vi "Navigation_Main_420.vi"() -> ()   [LabVIEW 2015]
uses:
  <vilib>/myRIO/Instrument Drivers/Onboard IO/PWM/typedefs/PWM Reference.ctl
  <vilib>/myRIO/Common/Instrument Driver Framework/Utilities/typedefs/myRIO Generic Hardware Reference.ctl
  <vilib>/myRIO/Common/Instrument Driver Framework/Utilities/typedefs/Hardware Version Enum.ctl
  <vilib>/myRIO/Common/Instrument Driver Framework/Utilities/typedefs/myRIO v1.0 Reference.ctl
  <vilib>/myRIO/Common/Instrument Driver Framework/Utilities/typedefs/Generic FPGA Reference.ctl
  <vilib>/myRIO/Common/Instrument Driver Framework/myRIO v1.0/PWM/typedefs/PWM Channels Enum.ctl
  <vilib>/myRIO/Instrument Drivers/Onboard IO/PWM/typedefs/PWM Configuration.ctl
  <vilib>/userdefined/High Color/nirio_resource_hc.ctl
  <vilib>/myRIO/Common/Instrument Driver Framework/myRIO v1.0/PWM/vis/myRIO v1.1 Open PWM.vi
  <vilib>/myRIO/Common/Instrument Driver Framework/Utilities/vis/Validate Channels.vi
  <vilib>/myRIO/Common/Instrument Driver Framework/myRIO v1.0/PWM/vis/myRIO v1.0 Reserve PWM.vi
  <vilib>/myRIO/Common/Instrument Driver Framework/myRIO v1.0/PWM/vis/myRIO v1.0 Build MUX Configuration PWM.vi
  <vilib>/myRIO/Common/Instrument Driver Framework/myRIO v1.0/Resource Manager/vis/myRIO v1.0 Reserve Channel List.vi
  <vilib>/myRIO/Common/Instrument Driver Framework/myRIO v1.0/Resource Manager/vis/myRIO v1.0 Create Configuration List.vi
  <vilib>/myRIO/Common/Instrument Driver Framework/myRIO v1.0/Resource Manager/vis/myRIO v1.0 Reserve Channel.vi
  <vilib>/myRIO/Common/Instrument Driver Framework/myRIO v1.0/Resource Manager/vis/myRIO v1.0 Unreserve Channel.vi
  <vilib>/myRIO/Common/Instrument Driver Framework/myRIO v1.0/Resource Manager/vis/myRIO v1.0 Build Mutex Name.vi
  <vilib>/FPGAPlugInAG/myRIO-1900/niLvFpga_Open_myRIO-1900.vi
  <vilib>/rvi/interface/common/dynamic/niFpgaDynamicAddResources.vi
  <vilib>/myRIO/Common/Instrument Driver Framework/Utilities/vis/FPGA Ref Manager.vi
  <vilib>/Utility/error.llb/Error Cluster From Error Code.vi
  <vilib>/myRIO/Common/Instrument Driver Framework/Utilities/vis/Ref Counter.vi
  <vilib>/rvi/errors/niLvFpgaAdjustHostInterfaceError.vi
  <vilib>/Utility/VariantDataType/GetNumericInfo.vi
  <vilib>/myRIO/Common/Instrument Driver Framework/myRIO v1.0/myRIO v1.1 Open.vi
  <vilib>/myRIO/Common/Instrument Driver Framework/Utilities/vis/IO Manager.vi
  <vilib>/myRIO/Common/Instrument Driver Framework/Utilities/vis/Configuration Manager.vi
  <vilib>/myRIO/Common/Instrument Driver Framework/myRIO v1.0/Resource Manager/vis/myRIO v1.0 Configure IO.vi
  <vilib>/myRIO/Common/Instrument Driver Framework/myRIO v1.0/myRIO v1.0 Close.vi
  <vilib>/myRIO/Common/Instrument Driver Framework/myRIO v1.0/PWM/vis/myRIO v1.0 Write PWM.vi
  <vilib>/addons/control/pid/pid.llb/PID (DBL).vi
  <vilib>/rvi/interface/nirviOpenFPGA/nirviOpenFPGA.xnode
  Navi/E/FPGA Bitfiles/NavigationProjec_FPGATarget2_FPGAMainNavigati_PWPHW8gwDxI.lvbitx
  <vilib>/rvi/interface/nirviReadWriteControl/nirviReadWriteControl.xnode
  <vilib>/myRIO/Instrument Drivers/Onboard IO/PWM/vis/myRIO PWM Open.xnode
  <vilib>/myRIO/Instrument Drivers/Onboard IO/PWM/PWM.lvlib
  <vilib>/myRIO/Instrument Drivers/Utilities/Utilities.lvlib
  NiFpgaLv.dll
  <vilib>/rvi/interface/Simulation/niFpgaSimulationCallBeginRW.vi
  <vilib>/addons/control/pid/NI_PID_pid.lvlib
panel:
  in  "start":dbl
  in  "end mining section":bool
  in  "frame":dbl format="%#_13g"
  in  "goal":dbl=10.0
  in  "first good x":dbl
  in  "drive 1 ft":dbl
  in  "end loop":bool
  out "stop switch":dbl
  in  "camera drop":dbl
  in  "derp":dbl
  in  "dead recon offset":dbl
  in  "last good x":dbl
  out "scale 2":dbl=1.0
  out "distance to goal":dbl
  out "loc_y":dbl
  out "loc_x":dbl
  out "loc_theta":dbl
  out "start y":dbl
  out "start angle":dbl=1.0
  out "start x":dbl=1.0
  in  "set start position":bool
  in  "R Min Linear Velocity (ft/s)  2":dbl=-2.0 format="%#_13g"
  in  "L Min Linear Velocity (ft/s) 9":dbl=-2.0 format="%#_13g"
  in  "R Max Linear Velocity (ft/s) 5":dbl=2.0 format="%#_13g"
  in  "L Max Linear Velocity (ft/s) 5":dbl=2.0 format="%#_13g"
  out "left wheels actual pwm":dbl
  in  "stop 3":bool
  out "left pwm":dbl(graph)
  out "dt out (s) 3":dbl format="%.3f"
  in  "output range 3":cluster{"output high":dbl, "output low":dbl}={"output high"=0.13333, "output low"=-0.13333} {"output low" format="%.6f"; "output high" format="%.5f"}
  in  "PID gains 3":T1={"proportional gain (Kc)"=0.002, "integral time (Ti, min)"=7e-07, "derivative time (Td, min)"=0.0} {"derivative time (Td, min)" format="%.8f"; "integral time (Ti, min)" format="%.8f"; "proportional gain (Kc)" format="%.8f"}
  out "desired pwm 2":dbl
  out "feedback 2":dbl
  out ".not. x? 3":bool
  out "Elapsed Time (s) 2":dbl caption="Elapsed Time (s)"
  out "right wheels actual pwm":dbl
  in  "stop 2":bool
  out "right pwm":dbl(graph)
  out "dt out (s) 2":dbl format="%.3f"
  in  "output range 2":cluster{"output high":dbl, "output low":dbl}={"output high"=0.13333, "output low"=-0.13333} {"output low" format="%.6f"; "output high" format="%.5f"}
  in  "PID gains 2":T1={"proportional gain (Kc)"=0.002, "integral time (Ti, min)"=7e-07, "derivative time (Td, min)"=0.0} {"derivative time (Td, min)" format="%.8f"; "integral time (Ti, min)" format="%.8f"; "proportional gain (Kc)" format="%.8f"}
  out "desired pwm":dbl
  out "feedback":dbl
  out ".not. x? 2":bool
  out "Elapsed Time (s)":dbl
  out "LF Rot Velocity (rot/s)":dbl
  out "LM Rot Velocity (rot/s)":dbl
  out "LR Rot Velocity (rot/s)":dbl
  out "RR Rot Velocity (rot/s)":dbl
  out "RM Linear Velocity (rot/s)":dbl
  out "RF Linear Velocity (rot/s)":dbl
  in  "Encoder Reset":bool
  out "SYS.SELECTA":u8 format="%08b"
  out "ENC.B_c.CNTR":i32
  out "ENC.B_b.CNTR":i32
  out "ENC.B_a.CNTR":i32
  out "ENC.A_c.CNTR":i32
  out "ENC.A_b.CNTR":i32
  out "ENC.A_a.CNTR":i32
  in  "R Min Linear Velocity (ft/s)":dbl=-2.0 format="%#_13g"
  in  "R Max Linear Velocity (ft/s)":dbl=2.0 format="%#_13g"
  in  "L Min Linear Velocity (ft/s)":dbl=-2.0 format="%#_13g"
  in  "L Max Linear Velocity (ft/s)":dbl=2.0 format="%#_13g"
  out "Current Rot Velocity (rot/s)":T2(graph)
  # "Motor Control Parameters"
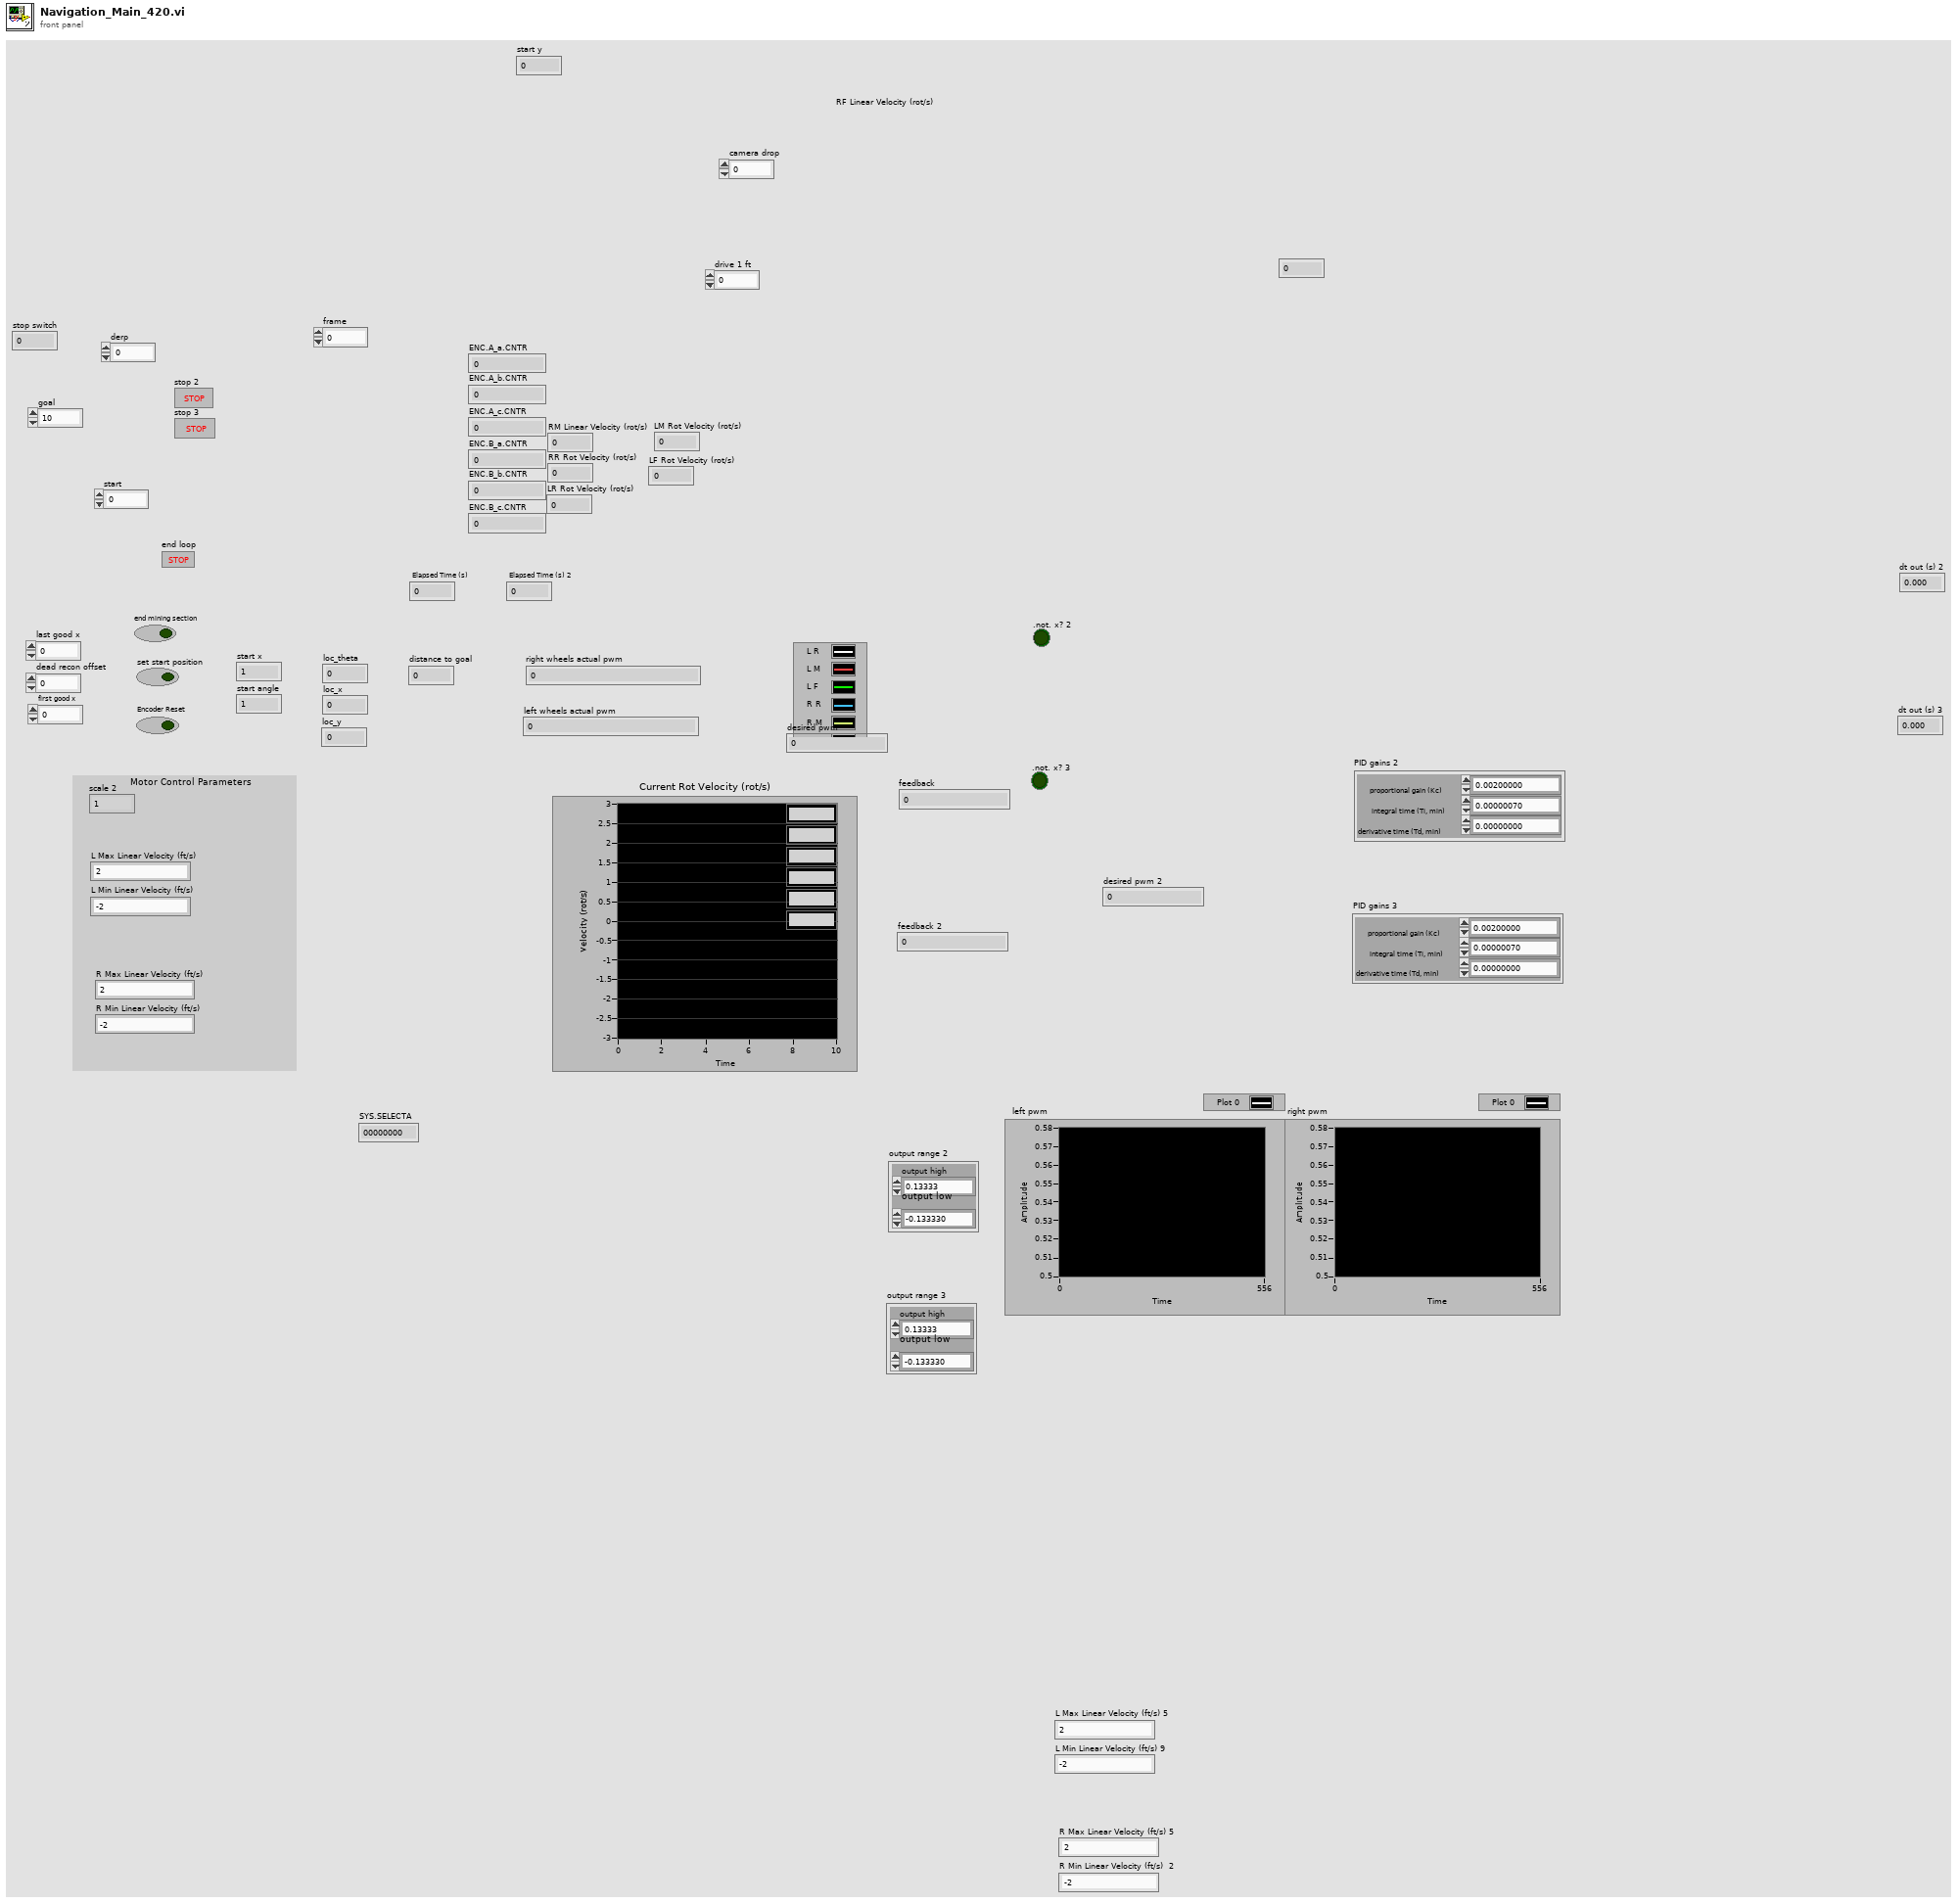
[diagram p1: front panel]
types:
  T1 = cluster{"proportional gain (Kc)":dbl, "integral time (Ti, min)":dbl, "derivative time (Td, min)":dbl}
  T2 = cluster{"Rotational Velocity (RPS)":dbl, "Rotational Velocity (RPS)":dbl, "Rotational Velocity (RPS)":dbl, "Rotational Velocity (RPS)":dbl, "Rotational Velocity (RPS)":dbl, "Rotational Velocity (RPS)":dbl}
  T3 = typedef "nirio_resource_hc.ctl" = tag
  T4 = typedef "Hardware Version Enum.ctl" = enum16{"Unknown", "myRIO-1900", "myRIO-1950", "roboRIO"}
  T5 = typedef "PWM.lvlib/PWM Reference.ctl" = cluster{"myRIO Reference":T6, "PWM Channels Enum":T9, "PWM Configuration":T10}
  T6 = typedef "myRIO Generic Hardware Reference.ctl" = cluster{"myRIO Model":T4, "myRIO Hardware Reference":T7}
  T7 = typedef "myRIO v1.0 Reference.ctl" = cluster{"Generic FPGA Reference":T8, "Allow multiple opens":bool}
  T8 = typedef "Generic FPGA Reference.ctl" = refnum<k20>
  T9 = typedef "PWM Channels Enum.ctl" = enum16{"Not Connected", "C/PWM0", "C/PWM1", "A/PWM0", "A/PWM1", "A/PWM2", "B/PWM0", "B/PWM1", "B/PWM2", "PWM/PWM0", "PWM/PWM1", "PWM/PWM2", "PWM/PWM3", "PWM/PWM4", "PWM/PWM5", "PWM/PWM6", "PWM/PWM7", "PWM/PWM8", "PWM/PWM9"}
  T10 = typedef "PWM.lvlib/PWM Configuration.ctl" = cluster{"Frequency":dbl, "Duty Cycle":dbl}
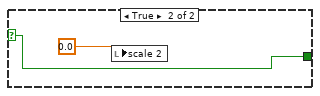
[diagram p3: hidden frame]
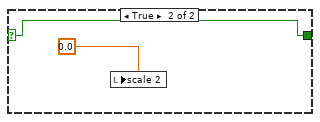
[diagram p4: hidden frame]
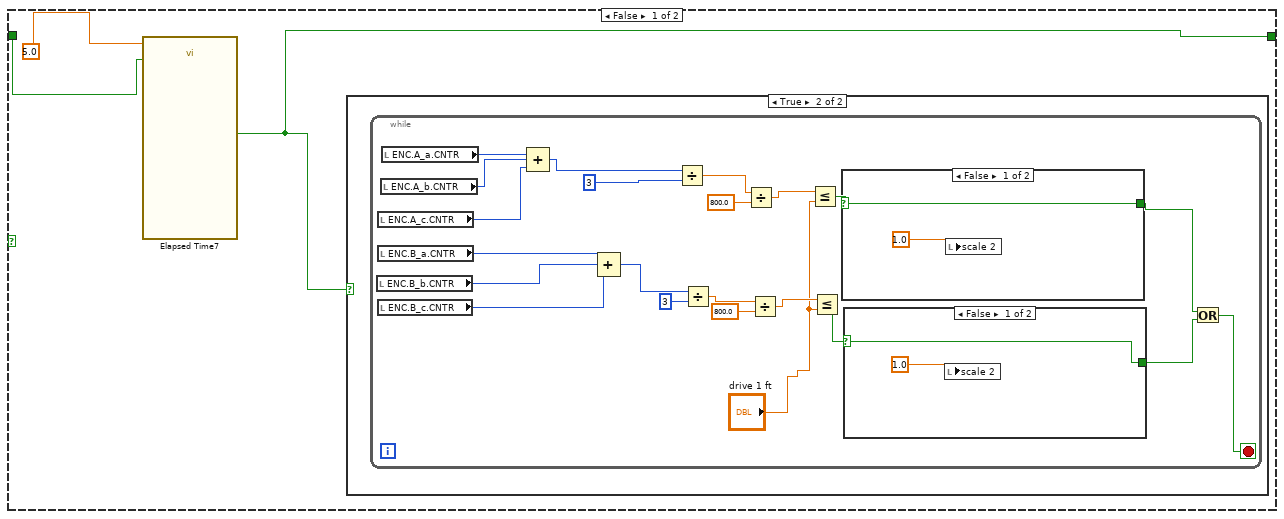
[diagram p5: hidden frame]
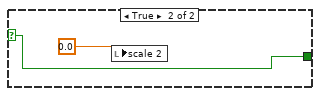
[diagram p7: hidden frame]
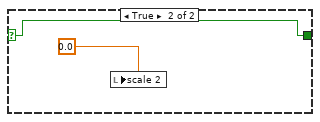
[diagram p8: hidden frame]
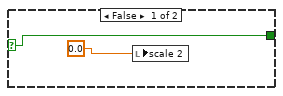
[diagram p9: hidden frame]
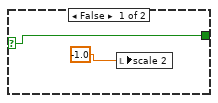
[diagram p10: hidden frame]
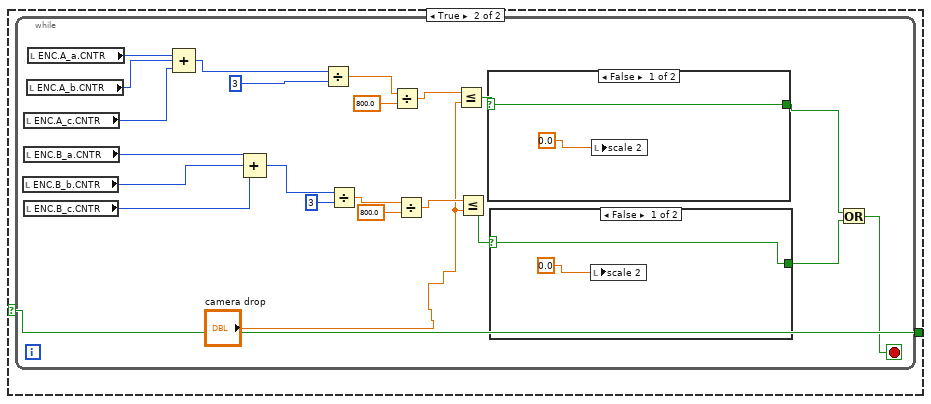
[diagram p11: hidden frame]
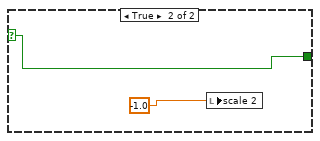
[diagram p12: hidden frame]
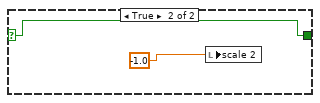
[diagram p13: hidden frame]
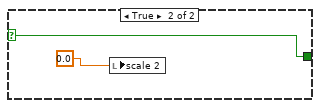
[diagram p14: hidden frame]
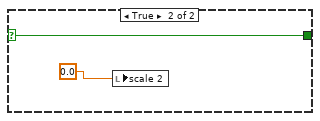
[diagram p15: hidden frame]
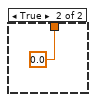
[diagram p17: hidden frame]
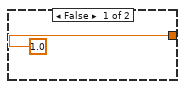
[diagram p18: hidden frame]
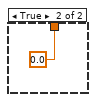
[diagram p19: hidden frame]
diagram:
  n1 = flat-sequence {
    tunnel: [w33] -> w30
    tunnel: [w33] -> w29
    tunnel: [w46] -> w28
    tunnel: [w61] -> w26
    tunnel: [w57] -> w24
    tunnel: [w56] -> w22
    tunnel: [w55] -> w20
    tunnel: [w54] -> w18
    tunnel: [w53] -> w16
    tunnel: ["L Max Linear Velocity (ft/s)"] -> w14
    tunnel: ["L Min Linear Velocity (ft/s)"] -> w12
    tunnel: ["R Max Linear Velocity (ft/s)"] -> w10
    tunnel: ["R Min Linear Velocity (ft/s)"] -> w8
    tunnel: [w48] -> w6
    tunnel: w30 -> [w47]
    tunnel: [w47] -> w4
    tunnel: w29 -> [w48]
    tunnel: [w46] -> w2
    tunnel: w28 -> [w187]
    tunnel: [w187] -> w27
    tunnel: w26 -> [w186]
    tunnel: [w186] -> w25
    tunnel: w24 -> [w185]
    tunnel: [w185] -> w23
    tunnel: w22 -> [w184]
    tunnel: [w184] -> w21
    tunnel: w20 -> [w183]
    tunnel: [w183] -> w19
    tunnel: w18 -> [w182]
    tunnel: [w182] -> w17
    tunnel: w16 -> [w181]
    tunnel: [w181] -> w15
    tunnel: w14 -> [w180]
    tunnel: [w180] -> w13
    tunnel: w12 -> [w179]
    tunnel: [w179] -> w11
    tunnel: w10 -> [w178]
    tunnel: [w178] -> w9
    tunnel: w8 -> [w177]
    tunnel: [w177] -> w7
    tunnel: w6 -> [w176]
    tunnel: [w176] -> w5
    tunnel: w4 -> [w175]
    tunnel: [w175] -> w3
    tunnel: w2 -> [w174]
    tunnel: [w174] -> w1
    tunnel: w27 -> [_]
    tunnel: w25 -> [w197]
    tunnel: w23 -> [w203]
    tunnel: w21 -> [w200]
    tunnel: w19 -> [w199]
    tunnel: w17 -> [w198]
    tunnel: w15 -> [w202]
    tunnel: w13 -> [_]
    tunnel: w11 -> [_]
    tunnel: w9 -> [_]
    tunnel: w7 -> [_]
    tunnel: w5 -> [w205]
    tunnel: w3 -> [w204]
    tunnel: w1 -> [w201]
    frame #0 {
      n2 = flat-sequence {
        tunnel: w34 -> [w39]
        tunnel: [w37] -> w36
        tunnel: w36 -> [w41]
        tunnel: [w41] -> w35
        tunnel: w35 -> [w44]
        tunnel: [w43] -> w33
        frame #0 {
          w38 = u8 32 ("SYS.SELECTA")
          w40 = u8 3 ("ENC.B_c.CNFG")
          n3 = xnode "Read/Write Control"("FPGA VI Reference In"=w39, "ENC.A_a.CNFG"=w40, "ENC.A_b.CNFG"=w40, "ENC.A_c.CNFG"=w40, "ENC.B_a.CNFG"=w40, "ENC.B_b.CNFG"=w40, "ENC.B_c.CNFG"=w40, "SYS.SELECTA"=w38, "SYS.SELECTB"=w38) -> ("FPGA VI Reference Out"=w37:refnum<k20>)  [unwired: 1 in, 1 out]
        }
        frame #1 {
          n4 = Wait (ms)(milliseconds to wait=u32 10) -> ()  [unwired: 1 out]
        }
        frame #2 {
          w45 = u8 1 ("ENC.B_c.CNFG")
          n5 = xnode "Read/Write Control"("FPGA VI Reference In"=w44, "ENC.A_a.CNFG"=w45, "ENC.A_b.CNFG"=w45, "ENC.A_c.CNFG"=w45, "ENC.B_a.CNFG"=w45, "ENC.B_b.CNFG"=w45, "ENC.B_c.CNFG"=w45) -> ("FPGA VI Reference Out"=w43:refnum<k20>)  [unwired: 1 in, 1 out]
        }
      }
      n6 = xnode "Open FPGA VI Reference"("resource name"=tag "RIO0") -> ("FPGA VI Reference Out"=w32:refnum<k20>)  [unwired: 1 in, 1 out]
      n7 = call <vilib>:"Set Custom Bitfile.vi"("Custom FPGA Reference In"=w32) -> ("Custom FPGA Reference Out"=w34:refnum<k20>)  [unwired: 9 in, 1 out]
    }
    frame #1 {
      w58 = 0.5 ("Duty Cycle")
      w46 = 333.333 ("Frequency [Hz]")
      w72 = tag "B/PWM2"  # Right rear ch
      w73 = tag "B/PWM0"  # Right mid ch
      w74 = tag "B/PWM1"  # Right front ch
      w75 = tag "A/PWM2"  # Left rear ch
      w76 = tag "A/PWM1"  # Left mid ch
      w77 = tag "A/PWM0"  # Left front ch
      n8 = xnode "Right  Front"("Channel Name"=w74) -> ("PWM Ref Out"=w68:T5)  [unwired: 2 in, 1 out]
      n9 = xnode "Right  Rear"("Channel Name"=w72) -> ("PWM Ref Out"=w66:T5)  [unwired: 2 in, 1 out]
      n10 = xnode "Left Front"("Channel Name"=w77) -> ("PWM Ref Out"=w71:T5)  [unwired: 2 in, 1 out]
      n11 = xnode "Right  Mid"("Channel Name"=w73) -> ("PWM Ref Out"=w67:T5)  [unwired: 2 in, 1 out]
      n12 = xnode "Left Rear"("Channel Name"=w75) -> ("PWM Ref Out"=w69:T5)  [unwired: 2 in, 1 out]
      n13 = xnode "Left Mid"("Channel Name"=w76) -> ("PWM Ref Out"=w70:T5)  [unwired: 2 in, 1 out]
      n14 = call <vilib>:"Set Frequency.vi"("Frequency [Hz]"=w46, "PWM Ref In"=w68) -> ("PWM Ref Out"=w62:T5)  [unwired: 7 in, 1 out]
      n15 = call <vilib>:"Set Frequency.vi"("Frequency [Hz]"=w46, "PWM Ref In"=w67) -> ("PWM Ref Out"=w63:T5)  [unwired: 7 in, 1 out]
      n16 = call <vilib>:"Set Frequency.vi"("Frequency [Hz]"=w46, "PWM Ref In"=w66) -> ("PWM Ref Out"=w64:T5)  [unwired: 7 in, 1 out]
      n17 = call <vilib>:"Set Frequency.vi"("Frequency [Hz]"=w46, "PWM Ref In"=w70) -> ("PWM Ref Out"=w59:T5)  [unwired: 7 in, 1 out]
      n18 = call <vilib>:"Set Frequency.vi"("Frequency [Hz]"=w46, "PWM Ref In"=w71) -> ("PWM Ref Out"=w65:T5)  [unwired: 7 in, 1 out]
      n19 = call <vilib>:"Set Frequency.vi"("Frequency [Hz]"=w46, "PWM Ref In"=w69) -> ("PWM Ref Out"=w60:T5)  [unwired: 7 in, 1 out]
      n20 = call <vilib>:"Set Duty Cycle.vi"("Duty Cycle"=w58, "PWM Ref In"=w62) -> ("PWM Ref Out"=w57:T5)  [unwired: 7 in, 1 out]
      n21 = call <vilib>:"Set Duty Cycle.vi"("Duty Cycle"=w58, "PWM Ref In"=w63) -> ("PWM Ref Out"=w56:T5)  [unwired: 7 in, 1 out]
      n22 = call <vilib>:"Set Duty Cycle.vi"("Duty Cycle"=w58, "PWM Ref In"=w64) -> ("PWM Ref Out"=w55:T5)  [unwired: 7 in, 1 out]
      n23 = call <vilib>:"Set Duty Cycle.vi"("Duty Cycle"=w58, "PWM Ref In"=w59) -> ("PWM Ref Out"=w54:T5)  [unwired: 7 in, 1 out]
      n24 = call <vilib>:"Set Duty Cycle.vi"("Duty Cycle"=w58, "PWM Ref In"=w65) -> ("PWM Ref Out"=w53:T5)  [unwired: 7 in, 1 out]
      n25 = call <vilib>:"Set Duty Cycle.vi"("Duty Cycle"=w58, "PWM Ref In"=w60) -> ("PWM Ref Out"=w61:T5)  [unwired: 7 in, 1 out]
    }
    frame #2 {
      n26 = while {
        stop <- w188 stop-if-true
        n27 = case shown="True" "set start position" {
          selector: "set start position" -> [_ w194]
          tunnel: [_ w194] -> w188
          frame False {
          }
          frame True {
            n28 = shared-variable "RT myRIO Target - Overlord\\Localization_Variables_r0.lvlib\\loc_x"() -> (→"start x":dbl)  [unwired: 1 in, 1 out]
            n29 = shared-variable "RT myRIO Target - Overlord\\Localization_Variables_r0.lvlib\\loc_y"() -> (→"start y":dbl)  [unwired: 1 in, 1 out]
            n30 = shared-variable "RT myRIO Target - Overlord\\Localization_Variables_r0.lvlib\\loc_theta"() -> (→"start angle":dbl)  [unwired: 1 in, 1 out]
            n31 = Wait (ms)(milliseconds to wait=u32 500) -> ()  [unwired: 1 out]
          }
        }
      }
    }
    frame #3 {
      (unwired) FALSE
      # "Uses quadrature encoder tick count to calculate rotational and linear velocity for a wheel."
      # "20ms loop delay to allow the encoder to travel far enough for a good update. 20ms provides 50Hz update rate to match motor PWM output rate."
      n32 = while {
        stop <- "end loop" stop-if-true
        n33 = flat-sequence {
          frame #0 {
            # "starting guess for offset is like 5 i guess"
            # "need to figure out which encoder is dead and divide by 2 instead of 3"
            # "start at bin and drive away some pre determined distance for cameras to track beacon"
            n34 = while {
              stop <- w210 stop-if-true
              n35 = local read "ENC.B_b.CNTR"() -> (w229:i32)
              n36 = local read "ENC.A_c.CNTR"() -> (w227:i32)
              n37 = local read "ENC.B_a.CNTR"() -> (w230:i32)
              n38 = local read "ENC.B_c.CNTR"() -> (w228:i32)
              n39 = local read "ENC.A_b.CNTR"() -> (w226:i32)
              n40 = local read "ENC.A_a.CNTR"() -> (w225:i32)
              n41 = Compound Arithmetic op=ADD(w225, w226, w227) -> (w224:i32)
              n42 = Compound Arithmetic op=ADD(w230, w229, w228) -> (w221:i32)
              n43 = Divide(x=w224, y=1) -> (x/y=w220:dbl)
              n44 = Divide(x=w221, y=1) -> (x/y=w219:dbl)
              n45 = Divide(x=w220, y=400.0) -> (x/y=w216:dbl)
              n46 = Divide(x=w219, y=400.0) -> (x/y=w215:dbl)
              n47 = Greater Or Equal?(x=w216, y="dead recon offset") -> (x >= y?=w213:bool)
              n48 = Greater Or Equal?(x=w215, y="dead recon offset") -> (x >= y?=w214:bool)
              n49 = case shown="False" w213 {
                selector: w213 -> [w235 w237]
                tunnel: [w235 w237] -> w212
                frame False {
                  n50 = local write "scale 2"(1.0) -> ()
                }
                frame True {
                  n51 = local write "scale 2"(0.0) -> ()
                }
              }
              n52 = case shown="False" w214 {
                selector: w214 -> [w231 w233]
                tunnel: [w231 w233] -> w211
                frame False {
                  n53 = local write "scale 2"(1.0) -> ()
                }
                frame True {
                  n54 = local write "scale 2"(0.0) -> ()
                }
              }
              n55 = Not And(1:w211, 2:w212) -> (0:w210:bool)
            }
            n56 = local write "frame"(1.0) -> ()
          }
          frame #1 {
            n57 = local write "frame"(2.0) -> ()
          }
          frame #2 {
            # "wait around till cameras give us the location"
            # "fuck so what if the camera doesnt find the beacons and we need to move some more?"
            n58 = while {
              shift-right: [w242] -> _
              shift-left: _ -> [w241]
              stop <- w243 stop-if-true
              n59 = shared-variable "RT myRIO Target - Overlord\\Localization_Variables_r0.lvlib\\loc_x"() -> (w245:dbl)  [unwired: 1 in, 1 out]
              n60 = Greater Or Equal?(x=w245, y=2.0) -> (x >= y?=w243:bool)
              n61 = case shown="True" w243 {
                tunnel: [w247 _] -> w242
                tunnel: w241 -> [w246 _]
                frame False {
                  n62 = call "Elapsed Time7"("Time Target (s)"=5.0 ("Elapsed Time (s)"), "Reset"=w246) -> ("Time has Elapsed"=w247:bool)  [unwired: 10 in, 7 out]
                  n63 = case shown="True" w247 {
                    frame False {
                    }
                    frame True {
                      n64 = while {
                        stop <- w250 stop-if-true
                        n65 = local read "ENC.B_b.CNTR"() -> (w269:i32)
                        n66 = local read "ENC.A_c.CNTR"() -> (w267:i32)
                        n67 = local read "ENC.B_a.CNTR"() -> (w270:i32)
                        n68 = local read "ENC.B_c.CNTR"() -> (w268:i32)
                        n69 = local read "ENC.A_b.CNTR"() -> (w266:i32)
                        n70 = local read "ENC.A_a.CNTR"() -> (w265:i32)
                        n71 = Compound Arithmetic op=ADD(w265, w266, w267) -> (w264:i32)
                        n72 = Compound Arithmetic op=ADD(w270, w269, w268) -> (w261:i32)
                        n73 = Divide(x=w264, y=3) -> (x/y=w260:dbl)
                        n74 = Divide(x=w261, y=3) -> (x/y=w259:dbl)
                        n75 = Divide(x=w260, y=800.0) -> (x/y=w256:dbl)
                        n76 = Divide(x=w259, y=800.0) -> (x/y=w255:dbl)
                        n77 = Less Or Equal?(x=w256, y="drive 1 ft") -> (x <= y?=w253:bool)
                        n78 = Less Or Equal?(x=w255, y="drive 1 ft") -> (x <= y?=w254:bool)
                        n79 = case shown="False" w253 {
                          selector: w253 -> [w275 w277]
                          tunnel: [w275 w277] -> w252
                          frame False {
                            n80 = local write "scale 2"(1.0) -> ()
                          }
                          frame True {
                            n81 = local write "scale 2"(0.0) -> ()
                          }
                        }
                        n82 = case shown="False" w254 {
                          selector: w254 -> [w271 w273]
                          tunnel: [w271 w273] -> w251
                          frame False {
                            n83 = local write "scale 2"(1.0) -> ()
                          }
                          frame True {
                            n84 = local write "scale 2"(0.0) -> ()
                          }
                        }
                        n85 = Or(x=w252, y=w251) -> (x .or. y?=w250:bool)
                      }
                    }
                  }
                }
                frame True {
                }
              }
            }
            n86 = local write "frame"(3.0) -> ()
          }
          frame #3 {
            n87 = local write "frame"(4.0) -> ()
          }
          frame #4 {
            # "drive from wherever the cameras kick in to the set goal"
            n88 = while {
              stop <- w282 continue-if-true
              n89 = shared-variable "RT myRIO Target - Overlord\\Localization_Variables_r0.lvlib\\loc_x"() -> (w287:dbl)  [unwired: 1 in, 1 out]
              n90 = Subtract(x=w287, y="goal") -> (x-y=w285:dbl)
              n91 = Less?(x=w285, y=0.0) -> (x < y?=w283:bool)
              n92 = case shown="True" w283 {
                selector: w283 -> [w288 w290]
                tunnel: [w288 w290] -> w282
                frame False {
                  n93 = local write "scale 2"(0.0) -> ()
                }
                frame True {
                  n94 = local write "scale 2"(1.0) -> ()
                }
              }
            }
            n95 = local write "Encoder Reset"(FALSE ("Encoder Reset")) -> ()
            n96 = local write "frame"(5.0) -> ()
          }
          frame #5 {
            # "park at goal and chill"
            n97 = call "Elapsed Time5"("Time Target (s)"=5.0 ("Elapsed Time (s)")) -> ()  [unwired: 11 in, 8 out]
            n98 = local write "frame"(6.0) -> ()
          }
          frame #6 {
            # "start mining and wait for it to finish"
            n99 = while {
              stop <- "end mining section" stop-if-true
            }
            n100 = local write "frame"(7.0) -> ()
          }
          frame #7 {
            # "move back to the deposition bin area untill cameras cut out"
            n101 = while {
              stop <- w299 stop-if-true
              n102 = shared-variable "RT myRIO Target - Overlord\\Localization_Variables_r0.lvlib\\loc_x"() -> (w300:dbl)  [unwired: 1 in, 1 out]
              n103 = Greater Or Equal?(x=w300, y=1.0) -> (x >= y?=w298:bool)
              n104 = call "Elapsed Time6"("Time Target (s)"=5.0, "Reset"=w298) -> ()  [unwired: 10 in, 8 out]
              n105 = case shown="False" w298 {
                selector: w298 -> [w303 w314]
                tunnel: [w303 w314] -> w299
                frame False {
                  n106 = while {
                    stop <- w304 stop-if-true
                    n107 = shared-variable "RT myRIO Target - Overlord\\Localization_Variables_r0.lvlib\\loc_x"() -> (w309:dbl)  [unwired: 1 in, 1 out]
                    n108 = Subtract(x=w309, y="start") -> (x-y=w307:dbl)
                    n109 = Less?(x=w307, y=0.0) -> (x < y?=w305:bool)
                    n110 = case shown="True" w305 {
                      selector: w305 -> [w310 w312]
                      tunnel: [w310 w312] -> w304
                      frame False {
                        n111 = local write "scale 2"(-1.0) -> ()
                      }
                      frame True {
                        n112 = local write "scale 2"(0.0) -> ()
                      }
                    }
                  }
                }
                frame True {
                  n113 = while {
                    stop <- w316 stop-if-true
                    n114 = local read "ENC.B_b.CNTR"() -> (w335:i32)
                    n115 = local read "ENC.A_c.CNTR"() -> (w333:i32)
                    n116 = local read "ENC.B_a.CNTR"() -> (w336:i32)
                    n117 = local read "ENC.B_c.CNTR"() -> (w334:i32)
                    n118 = local read "ENC.A_b.CNTR"() -> (w332:i32)
                    n119 = local read "ENC.A_a.CNTR"() -> (w331:i32)
                    n120 = Compound Arithmetic op=ADD(w331, w332, w333) -> (w330:i32)
                    n121 = Compound Arithmetic op=ADD(w336, w335, w334) -> (w327:i32)
                    n122 = Divide(x=w330, y=3) -> (x/y=w326:dbl)
                    n123 = Divide(x=w327, y=3) -> (x/y=w325:dbl)
                    n124 = Divide(x=w326, y=800.0) -> (x/y=w322:dbl)
                    n125 = Divide(x=w325, y=800.0) -> (x/y=w321:dbl)
                    n126 = Less Or Equal?(x=w322, y="camera drop") -> (x <= y?=w319:bool)
                    n127 = Less Or Equal?(x=w321, y="camera drop") -> (x <= y?=w320:bool)
                    n128 = case shown="False" w319 {
                      selector: w319 -> [w342 w344]
                      tunnel: [w342 w344] -> w318
                      frame False {
                        n129 = local write "scale 2"(0.0) -> ()
                      }
                      frame True {
                        n130 = local write "scale 2"(-1.0 ("y")) -> ()
                      }
                    }
                    n131 = case shown="False" w320 {
                      selector: w320 -> [w338 w340]
                      tunnel: [w338 w340] -> w317
                      frame False {
                        n132 = local write "scale 2"(0.0) -> ()
                      }
                      frame True {
                        n133 = local write "scale 2"(-1.0 ("y")) -> ()
                      }
                    }
                    n134 = Or(x=w318, y=w317) -> (x .or. y?=w316:bool)
                  }
                }
              }
            }
            n135 = local write "frame"(8.0) -> ()
            n136 = local write "Encoder Reset"(FALSE ("Encoder Reset")) -> ()
          }
          frame #8 {
            # "use encoders to get the rest of the way to the bin"
            n137 = while {
              stop <- w347 stop-if-true
              n138 = local read "ENC.B_b.CNTR"() -> (w366:i32)
              n139 = local read "ENC.A_c.CNTR"() -> (w364:i32)
              n140 = local read "ENC.B_a.CNTR"() -> (w367:i32)
              n141 = local read "ENC.B_c.CNTR"() -> (w365:i32)
              n142 = local read "ENC.A_b.CNTR"() -> (w363:i32)
              n143 = local read "ENC.A_a.CNTR"() -> (w362:i32)
              n144 = Compound Arithmetic op=ADD(w362, w363, w364) -> (w361:i32)
              n145 = Compound Arithmetic op=ADD(w367, w366, w365) -> (w358:i32)
              n146 = Divide(x=w361, y=2) -> (x/y=w357:dbl)
              n147 = Divide(x=w358, y=2) -> (x/y=w356:dbl)
              n148 = Divide(x=w357, y=400.0) -> (x/y=w353:dbl)
              n149 = Divide(x=w356, y=400.0) -> (x/y=w352:dbl)
              n150 = Greater Or Equal?(x=w353, y="derp") -> (x >= y?=w350:bool)
              n151 = Greater Or Equal?(x=w352, y="derp") -> (x >= y?=w351:bool)
              n152 = case shown="False" w350 {
                selector: w350 -> [w373 w375]
                tunnel: [w373 w375] -> w349
                frame False {
                  n153 = local write "scale 2"(-1.0 ("y")) -> ()
                }
                frame True {
                  n154 = local write "scale 2"(0.0) -> ()
                }
              }
              n155 = case shown="False" w351 {
                selector: w351 -> [w368 w371]
                tunnel: [w368 w371] -> w348
                frame False {
                  n156 = local write "scale 2"(-1.0 ("y")) -> ()
                }
                frame True {
                  n157 = local write "scale 2"(0.0) -> ()
                }
              }
              n158 = Or(x=w349, y=w348) -> (x .or. y?=w347:bool)
            }
            n159 = local write "frame"(9.0) -> ()
          }
          frame #9 {
            # "dump that shit"
            n160 = shared-variable "RT myRIO Target - Overlord\\Mining_Variables_r0.lvlib\\Stop"(FALSE ("Stop")) -> ()  [unwired: 1 in, 1 out]
            n161 = while {
              stop <- w378 stop-if-true
              n162 = shared-variable "RT myRIO Target - Overlord\\Mining_Variables_r0.lvlib\\Stop"() -> (w378:bool)  [unwired: 1 in, 1 out]
              n163 = shared-variable "RT myRIO Target - Overlord\\Mining_Variables_r0.lvlib\\Mine or Dump"(i16 -1 ("Mine or Dump")) -> ()  [unwired: 1 in, 1 out]
            }
            n164 = local write "frame"(10.0) -> ()
          }
        }
      }
      n165 = while {
        stop <- FALSE stop-if-true
        n166 = shared-variable "RT myRIO Target - Overlord\\Localization_Variables_r0.lvlib\\loc_x"() -> (w380:dbl)  [unwired: 1 in, 1 out]
        n167 = Greater Or Equal?(x=w380, y=1.0) -> (x >= y?=w381:bool)
        n168 = case shown="True" w381 {
          tunnel: w380 -> [_ w389]
          frame False {
          }
          frame True {
            n169 = local write "last good x"(w389) -> ()
          }
        }
        n170 = shared-variable "RT myRIO Target - Overlord\\Localization_Variables_r0.lvlib\\loc_x"() -> (w386:dbl)  [unwired: 1 in, 1 out]
        "loc_x" <- w386
        n171 = shared-variable "RT myRIO Target - Overlord\\Localization_Variables_r0.lvlib\\loc_y"() -> (→"loc_y":dbl)  [unwired: 1 in, 1 out]
        n172 = shared-variable "RT myRIO Target - Overlord\\Localization_Variables_r0.lvlib\\loc_theta"() -> (→"loc_theta":dbl)  [unwired: 1 in, 1 out]
        n173 = local read "goal"() -> (w385:dbl)
        n174 = Subtract(x=w386, y=w385) -> (x-y=→"distance to goal":dbl)
      }
      n175 = call "Tick Count"() -> ("Tick Count(uSec)"=w206:u32)
      n176 = while {
        tunnel: w205 -> [w455]
        stop <- FALSE stop-if-true
        n177 = xnode "Read/Write Control"("FPGA VI Reference In"=w455) -> ("SYS.SELECTA"=→"SYS.SELECTA":u8)  [unwired: 1 in, 2 out]
        n178 = xnode "Read/Write Control"("FPGA VI Reference In"=w455) -> ("ENC.A_a.CNTR"=→"ENC.A_a.CNTR":u32, "ENC.A_b.CNTR"=→"ENC.A_b.CNTR":u32, "ENC.A_c.CNTR"=→"ENC.A_c.CNTR":u32, "ENC.B_a.CNTR"=→"ENC.B_a.CNTR":u32, "ENC.B_b.CNTR"=→"ENC.B_b.CNTR":u32, "ENC.B_c.CNTR"=→"ENC.B_c.CNTR":u32)  [unwired: 1 in, 2 out]
        n179 = Wait (ms)(milliseconds to wait=u32 20) -> ()  [unwired: 1 out]
        n180 = case shown="True" "Encoder Reset" {
          tunnel: w455 -> [_ w465]
          frame False {
          }
          frame True {
            n181 = flat-sequence {
              tunnel: w465 -> [w470]
              tunnel: [w468] -> w467
              tunnel: w467 -> [w472]
              tunnel: [w472] -> w466
              tunnel: w466 -> [w475]
              tunnel: [w474] -> _
              frame #0 {
                w469 = u8 60 ("SYS.SELECTA")
                w471 = u8 3 ("ENC.B_c.CNFG")
                n182 = xnode "Read/Write Control"("FPGA VI Reference In"=w470, "ENC.A_a.CNFG"=w471, "ENC.A_b.CNFG"=w471, "ENC.A_c.CNFG"=w471, "ENC.B_a.CNFG"=w471, "ENC.B_b.CNFG"=w471, "ENC.B_c.CNFG"=w471, "SYS.SELECTA"=w469, "SYS.SELECTB"=w469) -> ("FPGA VI Reference Out"=w468:refnum<k20>)  [unwired: 1 in, 1 out]
              }
              frame #1 {
                n183 = Wait (ms)(milliseconds to wait=u32 10) -> ()  [unwired: 1 out]
              }
              frame #2 {
                w476 = u8 1 ("ENC.B_c.CNFG")
                n184 = xnode "Read/Write Control"("FPGA VI Reference In"=w475, "ENC.A_a.CNFG"=w476, "ENC.A_b.CNFG"=w476, "ENC.A_c.CNFG"=w476, "ENC.B_a.CNFG"=w476, "ENC.B_b.CNFG"=w476, "ENC.B_c.CNFG"=w476) -> ("FPGA VI Reference Out"=w474:refnum<k20>)  [unwired: 1 in, 1 out]
              }
            }
          }
        }
      }
      n185 = while {
        tunnel: w202 -> [w416]
        tunnel: [w417] -> _
        tunnel: w201 -> [w404]
        shift-right: [w403] -> _
        shift-left: _ -> [w412]
        shift-right: [w390] -> _
        shift-left: TRUE ("stop 3") -> [w397]
        tunnel: [w404] -> _
        tunnel: w198 -> [w406]
        tunnel: w197 -> [w405]
        stop <- "stop 3" stop-if-true
        w391 = -0.08 ("y")
        # "*****\n\n(true is supposed\nto be 0)"
        n186 = local read "scale 2"() -> (w392:dbl)
        n187 = local read "stop switch"() -> (w393:dbl)
        n188 = Multiply(x=w392, y=w391) -> (x*y=w402:dbl)
        n189 = Add(x=0.5, y=w391) -> (x+y=→"desired pwm 2":dbl)
        n190 = call "Elapsed Time2"("Reset"=w397) -> ("Elapsed Time (s)"=w396:dbl, "Time has Elapsed"=w400:bool)  [unwired: 11 in, 6 out]
        "Elapsed Time (s) 2" <- w396
        n191 = Multiply(x=w402, y=w393) -> (x*y=w401:dbl)
        n192 = Not(x=w400) -> (.not. x?=w410:bool)
        ".not. x? 3" <- w410
        n193 = Greater Or Equal?(x=w396, y=4.0) -> (x >= y?=w390:bool)
        n194 = case shown="False" w390 {
          tunnel: [1.0 0.0] -> w398
          frame False {
          }
          frame True {
          }
        }
        n195 = Multiply(x=w401, y=w398) -> (x*y=w399:dbl)
        n196 = call-poly <vilib>:"PID.vi"("reinitialize? (F)"=w410, "output range"="output range 3", "PID gains"="PID gains 3", "process variable"=w412, "setpoint"=w399) -> ("dt out (s)"=→"dt out (s) 3":dbl, "output"=w403:dbl)  [unwired: 5 in]
        n197 = Add(x=0.5, y=w403) -> (x+y=w394:dbl)
        "left wheels actual pwm" <- w394
        "left pwm" <- w394
        n198 = call <vilib>:"Set Duty Cycle and Frequency.vi"("Frequency [Hz]"=w404, "Duty Cycle"=w394, "PWM Ref In"=w416) -> ("PWM Ref Out"=w417:T5)  [unwired: 6 in, 1 out]
        n199 = call <vilib>:"Set Duty Cycle and Frequency.vi"("Frequency [Hz]"=w404, "Duty Cycle"=w394, "PWM Ref In"=w406) -> ()  [unwired: 6 in, 2 out]
        n200 = call <vilib>:"Set Duty Cycle and Frequency.vi"("Frequency [Hz]"=w404, "Duty Cycle"=w394, "PWM Ref In"=w405) -> ()  [unwired: 6 in, 2 out]
        "feedback 2" <- w412
      }
      n201 = while {
        tunnel: w203 -> [w448]
        tunnel: [w449] -> _
        tunnel: [w436] -> _
        shift-right: [w435] -> _
        shift-left: _ -> [w444]
        shift-right: [w422] -> _
        shift-left: TRUE ("stop 2") -> [w430]
        tunnel: w201 -> [w436]
        tunnel: w200 -> [w438]
        tunnel: w199 -> [w437]
        stop <- "stop 2" stop-if-true
        # "******"
        n202 = local read "scale 2"() -> (w424:dbl)
        n203 = Multiply(x=w424, y=-0.08) -> (x*y=w434:dbl)
        n204 = local read "stop switch"() -> (w425:dbl)
        n205 = Add(x=0.5, y=w434) -> (x+y=→"desired pwm":dbl)
        n206 = call "Elapsed Time"("Reset"=w430) -> ("Elapsed Time (s)"=w429:dbl, "Time has Elapsed"=w427:bool)  [unwired: 11 in, 6 out]
        "Elapsed Time (s)" <- w429
        n207 = Multiply(x=w434, y=w425) -> (x*y=w433:dbl)
        n208 = Not(x=w427) -> (.not. x?=w442:bool)
        ".not. x? 2" <- w442
        n209 = Greater Or Equal?(x=w429, y=4.0) -> (x >= y?=w422:bool)
        n210 = case shown="False" w422 {
          tunnel: [1.0 0.0] -> w431
          frame False {
          }
          frame True {
          }
        }
        n211 = Multiply(x=w433, y=w431) -> (x*y=w432:dbl)
        n212 = call-poly <vilib>:"PID.vi"("reinitialize? (F)"=w442, "output range"="output range 2", "PID gains"="PID gains 2", "process variable"=w444, "setpoint"=w432) -> ("dt out (s)"=→"dt out (s) 2":dbl, "output"=w435:dbl)  [unwired: 5 in]
        n213 = Add(x=0.5, y=w435) -> (x+y=w426:dbl)
        "right wheels actual pwm" <- w426
        "right pwm" <- w426
        n214 = call <vilib>:"Set Duty Cycle and Frequency.vi"("Frequency [Hz]"=w436, "Duty Cycle"=w426, "PWM Ref In"=w448) -> ("PWM Ref Out"=w449:T5)  [unwired: 6 in, 1 out]
        n215 = call <vilib>:"Set Duty Cycle and Frequency.vi"("Frequency [Hz]"=w436, "Duty Cycle"=w426, "PWM Ref In"=w437) -> ()  [unwired: 6 in, 2 out]
        n216 = call <vilib>:"Set Duty Cycle and Frequency.vi"("Frequency [Hz]"=w436, "Duty Cycle"=w426, "PWM Ref In"=w438) -> ()  [unwired: 6 in, 2 out]
        n217 = local read "Encoder Reset"() -> (w420:bool)
        n218 = case shown="True" w420 {
          tunnel: [1.0 0.0] -> w421
          frame False {
          }
          frame True {
          }
        }
        "stop switch" <- w421
        "feedback" <- w444
      }
      n219 = while {
        shift-right: [w495] -> _
        shift-left: _ -> [w494]
        shift-right: [w492] -> _
        shift-left: w206 -> [w491]
        tunnel: w204 -> [w502]
        stop <- FALSE stop-if-true
        n220 = xnode "Read/Write Control"("FPGA VI Reference In"=w502) -> ("ENC.A_a.CNTR"=w501:u32, "ENC.A_b.CNTR"=w500:u32, "ENC.A_c.CNTR"=w499:u32, "ENC.B_a.CNTR"=w498:u32, "ENC.B_b.CNTR"=w497:u32, "ENC.B_c.CNTR"=w496:u32)  [unwired: 1 in, 2 out]
        n221 = call "Wait"("Count(mSec)"=u32 20) -> ()  [unwired: 1 out]
        n222 = Build Array(w501, w500, w499, w498, w497, w496) -> (w495:u32[])
        n223 = Subtract(x=w495, y=w494) -> (x-y=w493:u32[])
        n224 = call "Tick Count2"() -> ("Tick Count(uSec)"=w492:u32)
        n225 = Index Array(array=w493) -> (element #1=w490:u32, element #2=w489:u32, element #3=w488:u32, element #4=w487:u32, element #5=w486:u32, element #6=w485:u32)  [unwired: 6 in]
        n226 = Subtract(x=w492, y=w491) -> (x-y=w484:u32)
        n227 = call "Encoder-Velocity_Conversion (SubVI).vi"("delta  Encoder Count"=w489, "dt (uSec)"=w484) -> ("Rotational Velocity (RPS)"=w479:dbl)  [unwired: 7 in, 2 out]
        "LM Rot Velocity (rot/s)" <- w479
        n228 = call "Encoder-Velocity_Conversion (SubVI).vi"("delta  Encoder Count"=w488, "dt (uSec)"=w484) -> ("Rotational Velocity (RPS)"=w478:dbl)  [unwired: 7 in, 2 out]
        "LF Rot Velocity (rot/s)" <- w478
        n229 = call "Encoder-Velocity_Conversion (SubVI).vi"("delta  Encoder Count"=w490, "dt (uSec)"=w484) -> ("Rotational Velocity (RPS)"=w480:dbl)  [unwired: 7 in, 2 out]
        "LR Rot Velocity (rot/s)" <- w480
        n230 = call "Encoder-Velocity_Conversion (SubVI).vi"("delta  Encoder Count"=w487, "dt (uSec)"=w484) -> ("Rotational Velocity (RPS)"=w477:dbl)  [unwired: 7 in, 2 out]
        "RR Rot Velocity (rot/s)" <- w477
        n231 = call "Encoder-Velocity_Conversion (SubVI).vi"("delta  Encoder Count"=w486, "dt (uSec)"=w484) -> ("Rotational Velocity (RPS)"=w481:dbl)  [unwired: 7 in, 2 out]
        "RM Linear Velocity (rot/s)" <- w481
        n232 = call "Encoder-Velocity_Conversion (SubVI).vi"("delta  Encoder Count"=w485, "dt (uSec)"=w484) -> ("Rotational Velocity (RPS)"=w482:dbl)  [unwired: 7 in, 2 out]
        "RF Linear Velocity (rot/s)" <- w482
        n233 = Bundle("Rotational Velocity (RPS)"=w480, "Rotational Velocity (RPS)"=w479, "Rotational Velocity (RPS)"=w478, "Rotational Velocity (RPS)"=w477, "Rotational Velocity (RPS)"=w481, "Rotational Velocity (RPS)"=w482) -> (→"Current Rot Velocity (rot/s)":T2)  [unwired: 1 in]
      }
    }
  }
